vi "PH_SHS_Analysis.ProcCases.vi"(0 "i ref in":refnum<vi>, 1 "selector":string, 2 "Data":T2, 3 "call cluster":T3={"Object"="", "Selector"="", "CallType"=enum."synchronous", "Async Object"="", "Async Selector"="", "Data Descriptor"="", "Data"=[], "Error #"=0, "Expire"=0}, 5 "error in (no error)":errorcluster) -> (14 "i ref out":refnum<vi>, 17 "answer cluster":T3={"Object"="", "Selector"="", "CallType"=enum."synchronous", "Async Object"="", "Async Selector"="", "Data Descriptor"="", "Data"=[], "Error #"=0, "Expire"=0}, 19 "error out":errorcluster)   [LabVIEW 2014, in "PH_SHS_Analysis.lvlib"]
doc: "This method is called by a process from within the default case in the event loop. The methods of a class that are linked to events will be called from THIS method. Add your code here."
uses:
  PH_SHS_Analysis.lvlib
  CS_Core/CSSystem/CoreDefs/CoreDefs.call_type.ctl
  CS_Core/BaseProcess/BaseProcess.descriptor string definition.ctl
  CS_Core/CSSystem/CoreDefs/CoreDefs.rawDataType.ctl
  CSlibraries-extern/shs/SHS_Analysis/SHS_DeviceConfig.ctl
  CS_Core/CSSystem/CoreLib/CoreLib.string 2 byte array.vi
  CS_Core/CSSystem/CoreLib/CoreLib.byte array 2 short.vi
  CS_Core/CSSystem/CoreLib/CoreLib.byte array 2 string.vi
  CS_Core/CSSystem/CoreLib/CoreLib.byte array 2 double.vi
  CS_Core/BaseProcess/BaseProcess.lvlib
  CS_Core/CSSystem/CoreLib/CoreLib.lvlib
  CS_Core/CAEObj/CAEObj.lvlib
  PH_Basics/PH_PSDBWriter/PH_PSDBWriter.lvlib
  PH_Basics/PH_Common/PH_Common.lvlib
  CSlibraries-extern/shs/SHS_Analysis/SHS_Analysis.lvlib
  PH_Basics/PH_Img_BaseClass/PH_Img_BaseClass.lvlib
  PH_Basics/PH_Cam_BaseClass/PH_Cam_BaseClass.lvlib
panel:
  in  "SHS Device Config":T1 {"wavelength [m]" format="%#_6p"; "pixel size [m/px]" format="%#_6p"; "focal length [m]" format="%#_6p"}
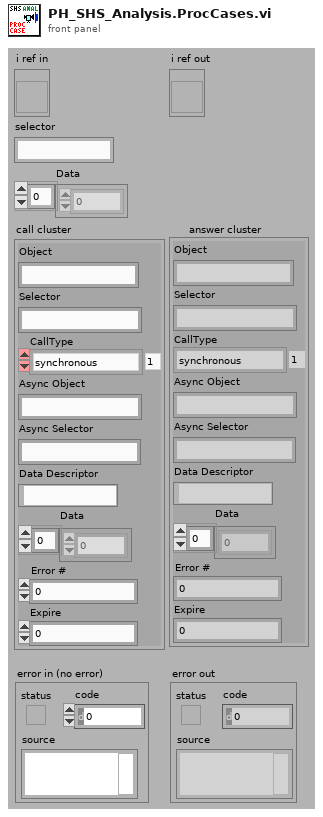
[diagram p1: front panel]
types:
  T1 = typedef "SHS_Analysis.lvlib/SHS_DeviceConfig.ctl" = cluster{"focal length [m]":dbl, "pixel size [m/px]":dbl, "wavelength [m]":dbl}
  T2 = typedef "CoreDefs.rawDataType.ctl" = i8[]
  T3 = typedef "CoreDefs.call_type.ctl" = cluster{"Object":string, "Selector":string, "CallType":enum16{"simple", "synchronous", "asynchronous"}, "Async Object":string, "Async Selector":string, "Data Descriptor":T4, "Data":T2, "Error #":i32, "Expire":u32}
  T4 = typedef "BaseProcess.lvlib/BaseProcess.descriptor string definition.ctl" = string
  T5 = cluster{"Cam ID":string, "Gain":dbl, "Brightness":dbl, "Shutter":dbl, "Cam Error":bool, "Mode":i32}
  T6 = enum8{"Enabled", "Disabled", "Disabled and Grayed Out"}
  T7 = typedef "PH_PSDBWriter.lvlib/PH_PSDBWriter.PHELIX-Subsystems.ctl" = i32
  T8 = typedef "PH_Cam_BaseClass.lvlib/PH_Cam_BaseClass.Settings.ctl" = cluster{"Cam ID":string, "Gain":dbl, "Brightness":dbl, "Shutter":dbl, "Mode":i32}
  T9 = typedef "PH_Img_BaseClass.lvlib/PH_Img_BaseClass.i attribute.ctl" = cluster{"GUI Refs":T10, "Timeout Image [ms]":i32, "Default Periodic Period [ms]":i32, "Camera":cluster{"Instancename":string, "Notifier":refnum<notifier>}, "Palette":T11, "Cam Settings":cluster{"Cam ID":string, "Gain":dbl, "Brightness":dbl, "Shutter":dbl, "Cam Info Failure":bool, "Mode":i32}}
  T10 = typedef "PH_Img_BaseClass.lvlib/PH_Img_BaseClass.GUI Refs.ctl" = cluster{"Timeout":refnum<vi>, "Image":refnum<vi>, "Palette":refnum<vi>, "Timeout Set":refnum<vi>}
  T11 = typedef "PH_Img_BaseClass.lvlib/PH_Img_BaseClass.Palette.ctl" = i32
  T12 = typedef "PH_SHS_Analysis.lvlib/PH_SHS_Analysis.i attribute.ctl" = cluster{"GUI Refs":cluster{"Delete":refnum<vi>, "Global On":refnum<vi>, "Cam Source":refnum<vi>, "Calibration Data File":refnum<vi>, "Calibration status":refnum<vi>, "Show overlay":refnum<vi>, "SHS Device Config":refnum<vi>, "Result":refnum<vi>, "Consider Tilt":refnum<vi>, "Working Reference":refnum<vi>, "Remove Tilt":refnum<vi>, "Take Cali  Reference":refnum<vi>, "Publishing Data Status":refnum<vi>, "Calibration Data":refnum<vi>}, "Calibration":cluster{"Status":T13, "Data":T14, "File":path}, "Result":T19, "Image":T22, "SHS Device Config":T1, "Show Overlay":bool, "GradientZernikeMatrix":dbl[][], "Consider Tilt":bool, "Working Reference":T15, "Zernicke Service ID":i32, "PSDB Image":T22}
  T13 = typedef "PH_StatusHandler.lvlib/PH_StatusHandler.Status.ctl" = i16
  T14 = typedef "PH_SHS_Analysis_Calibrator.lvlib/PH_SHS_Analysis_Calibrator.Analysis Calibration Data.ctl" = cluster{"Date":string, "Time":string, "Cam Settings":cluster{"Cam ID":string, "Gain":dbl, "Brightness":dbl, "Shutter":dbl, "Cam Error":bool, "Mode":i32}, "SHS Reference Result":T15, "Pixel Size":dbl, "MLA Pitch":dbl, "Method":enum16{"automatic", "manual"}, "Calibration Data calculated":bool, "No Problems at calculation?":bool, "error out":errorcluster}
  T15 = typedef "SHS_Common.lvlib/SHSReference.ctl" = cluster{"Reference":T16[][], "Lens Array Pitch [px]":dbl}
  T16 = typedef "SHS_Common.lvlib/ReferencePoint.ctl" = cluster{"Rect":T17, "Point":T18}
  T17 = typedef "SHS_Common.lvlib/Rectangle.ctl" = cluster{"Left":i32, "Top":i32, "Right":i32, "Bottom":i32}
  T18 = typedef "SHS_Common.lvlib/Point.ctl" = cluster{"x":dbl, "y":dbl, "valid?":bool, "weight":dbl}
  T19 = typedef "PH_SHS_Analysis.lvlib/PH_SHS_Analysis.Result.ctl" = cluster{"Time Stamp":timestamp, "Zernike Coefficients":T20, "PtV [lambda]":dbl, "Shifts":T21, "Measurement Quality":cluster{dbl, dbl, dbl}, "Measurement valid?":bool}
  T20 = typedef "PH_SHS_Analysis.lvlib/PH_SHS_Analysis.Zernike Coefficients.ctl" = cluster{"Tilt x":dbl, "Tilt y":dbl, "Defocus":dbl, "Astig 0°":dbl, "Astig 45°":dbl, "Coma x":dbl, "Coma y":dbl, "Spherical":dbl, "Trefoil 0°":dbl, "Trefoil 30°":dbl, "2nd Astig 0°":dbl, "2nd Astig 45°":dbl, "2nd Coma x":dbl, "2nd Coma y":dbl, "2nd Spherical":dbl}
  T21 = typedef "SHS_Common.lvlib/Shifts.ctl" = T18[][]
  T22 = typedef "IMAQ Image.ctl" = refnum<image>
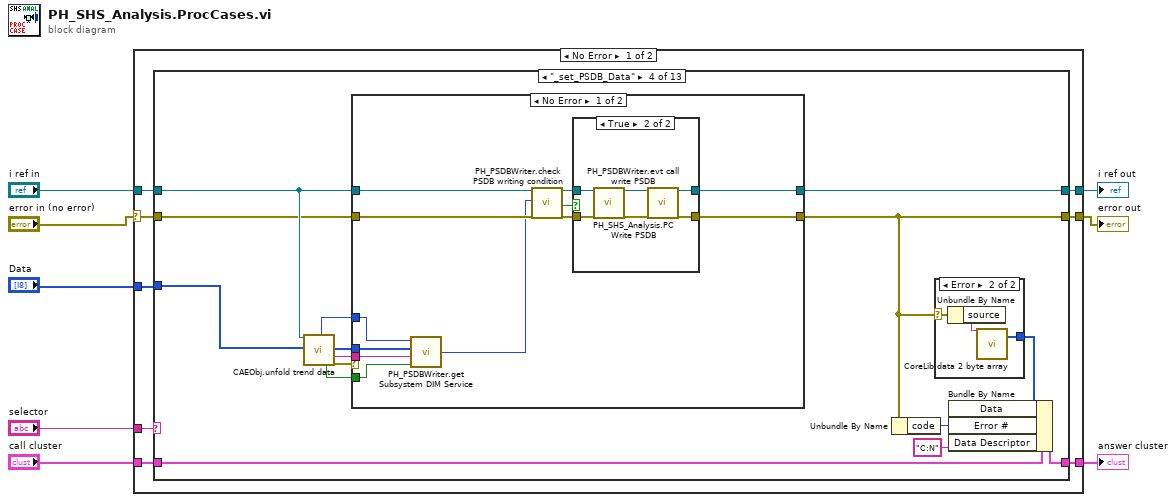
[diagram p0: block diagram]
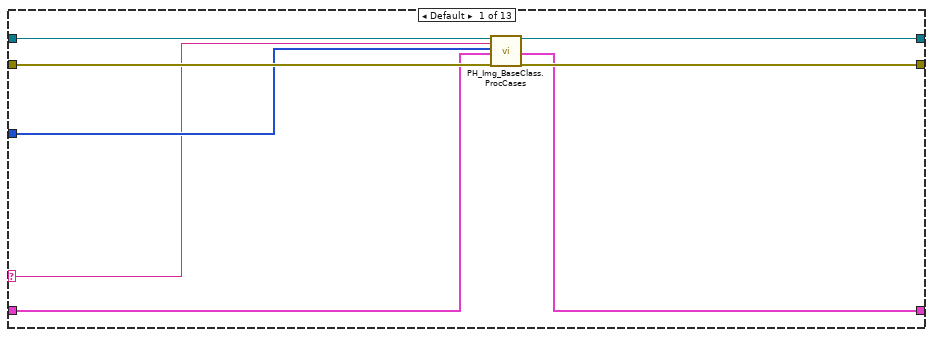
[diagram p2: hidden frame]
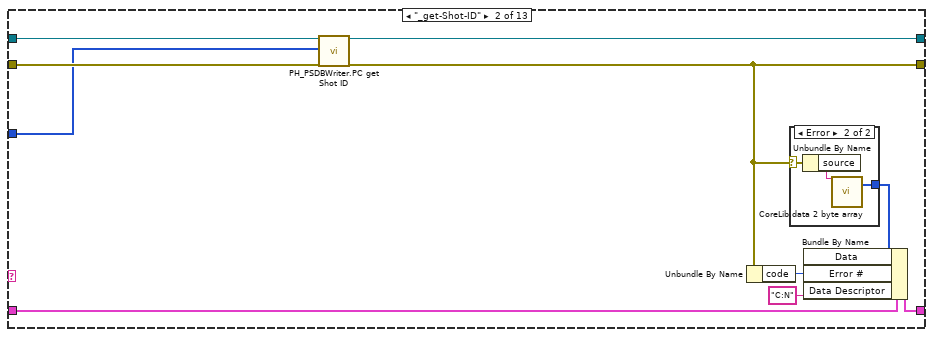
[diagram p3: hidden frame]
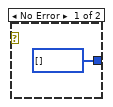
[diagram p4: hidden frame]
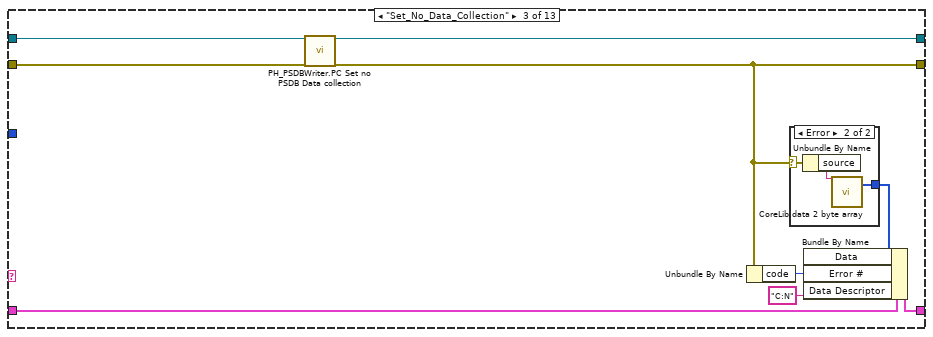
[diagram p5: hidden frame]
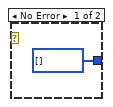
[diagram p6: hidden frame]
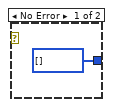
[diagram p9: hidden frame]
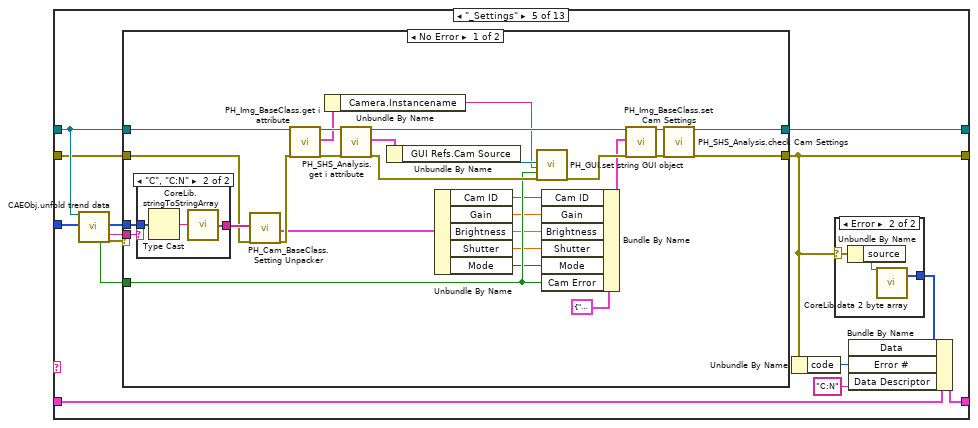
[diagram p10: hidden frame]
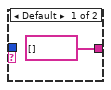
[diagram p11: hidden frame]
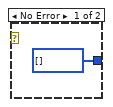
[diagram p13: hidden frame]
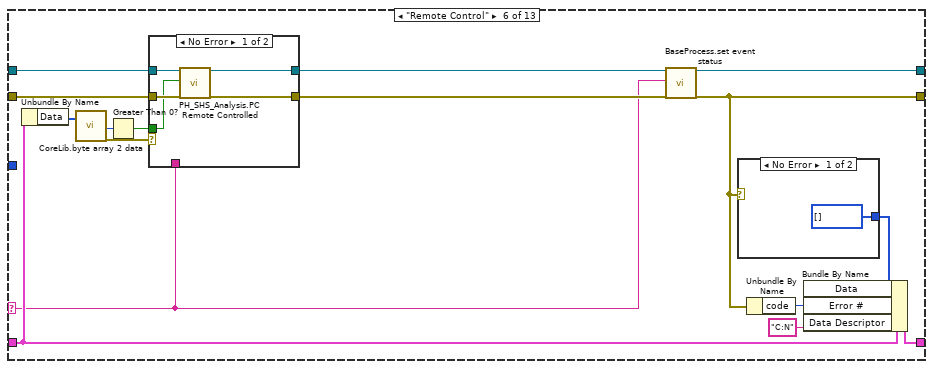
[diagram p14: hidden frame]
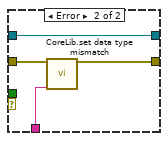
[diagram p15: hidden frame]
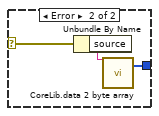
[diagram p16: hidden frame]
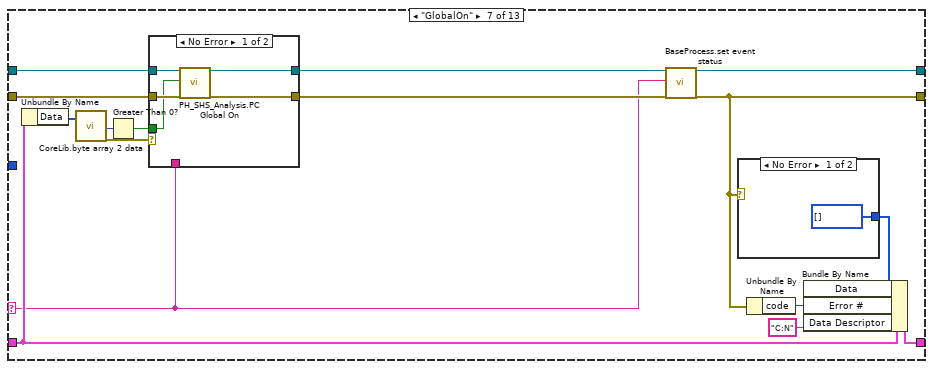
[diagram p17: hidden frame]
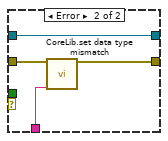
[diagram p18: hidden frame]
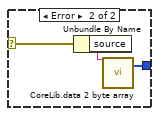
[diagram p19: hidden frame]
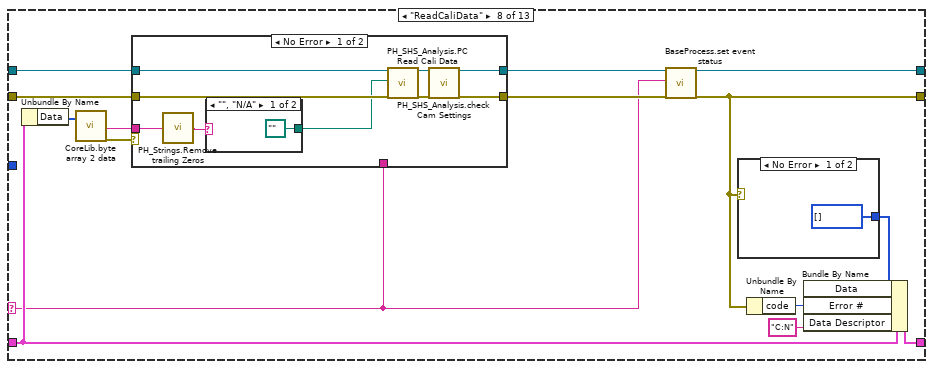
[diagram p20: hidden frame]
diagram:
  n1 = case shown="No Error" "error in (no error)" {
    selector: "error in (no error)" -> [w9 w456]
    tunnel: "selector" -> [w16 _]
    tunnel: [w15 w457] -> w7
    tunnel: "Data" -> [w14 _]
    tunnel: "call cluster" -> [w13 w457]
    tunnel: "i ref in" -> [w12 w458]
    tunnel: [w11 w458] -> w3
    tunnel: [w10 w456] -> w2
    frame No Error {
      n2 = case shown="\"_set_PSDB_Data\"" w16 {
        selector: w16 -> [w18 _ _ _ _ w145 w174 w204 w246 w293 w330 w374 w425]
        tunnel: w14 -> [w19 w25 _ w52 w97 _ _ _ _ _ _ _ _]
        tunnel: w12 -> [w17 w29 w41 w56 w96 w149 w178 w208 w245 w292 w335 w379 w430]
        tunnel: [w24 w27 w40 w54 w94 w156 w185 w213 w249 w296 w340 w384 w434] -> w11
        tunnel: w13 -> [w20 w33 w46 w65 w105 w148 w177 w207 w247 w294 w331 w375 w426]
        tunnel: [w21 w32 w45 w64 w104 w159 w188 w216 w252 w299 w343 w387 w437] -> w15
        tunnel: w9 -> [w23 w28 w42 w55 w95 w150 w179 w209 w244 w291 w334 w378 w429]
        tunnel: [w22 w26 w39 w53 w93 w157 w186 w214 w250 w297 w341 w385 w435] -> w10
        frame Default {
          n3 = call "PH_Img_BaseClass.ProcCases.vi"("i ref in"=w17, "selector"=w18, "Data"=w19, "call cluster"=w20, "error in (no error)"=w23) -> ("i ref out"=w24:refnum<vi>, "answer cluster"=w21:T3, "error out"=w22:errorcluster)  [unwired: 12 in]
        }
        frame "_get-Shot-ID" {
          n4 = call "PH_PSDBWriter.PC get Shot ID.vi"("i ref in"=w29, "Data"=w25, "error IO"=w28) -> ("i ref in"=w27:refnum<vi>, "error IO"=w26:errorcluster)  [unwired: 15 in]
          n5 = Unbundle By Name(w26) -> ("code"=w34:i32)
          n6 = case shown="Error" w26 {
            selector: w26 -> [_ w38]
            tunnel: [T2 [] ("byteArray out") w37] -> w31
            frame No Error {
            }
            frame Error {
              n7 = Unbundle By Name(w38) -> ("source"=w36:string)
              n8 = call-poly "CoreLib.data 2 byte array.vi"("string"=w36) -> ("byteArray out"=w37:T2)  [unwired: 18 in]
            }
          }
          n9 = Bundle By Name(cluster=w33, "Data"=w31, "Error #"=w34, "Data Descriptor"="C:N") -> (w32:T3)
        }
        frame "Set_No_Data_Collection" {
          n10 = call "PH_PSDBWriter.PC Set no PSDB Data collection.vi"("i ref in"=w41, "error IO"=w42) -> ("i ref out"=w40:refnum<vi>, "error out"=w39:errorcluster)  [unwired: 16 in]
          n11 = Unbundle By Name(w39) -> ("code"=w47:i32)
          n12 = case shown="Error" w39 {
            selector: w39 -> [_ w51]
            tunnel: [T2 [] ("byteArray out") w50] -> w44
            frame No Error {
            }
            frame Error {
              n13 = Unbundle By Name(w51) -> ("source"=w49:string)
              n14 = call-poly "CoreLib.data 2 byte array.vi"("string"=w49) -> ("byteArray out"=w50:T2)  [unwired: 18 in]
            }
          }
          n15 = Bundle By Name(cluster=w46, "Data"=w44, "Error #"=w47, "Data Descriptor"="C:N") -> (w45:T3)
        }
        frame "_set_PSDB_Data" {
          n16 = call "CAEObj.unfold trend data.vi"("i ref in"=w56, "raw trend data"=w52) -> ("quality"=w57:i32, "no link"=w60:bool, "data"=w58:i8[], "typeDescriptor"=w59:string, "error out"=w61:errorcluster)  [unwired: 9 in, 4 out]
          n17 = case shown="No Error" w61 {
            tunnel: w55 -> [w78 w88]
            tunnel: [w77 w87] -> w54
            tunnel: [w76 w88] -> w53
            tunnel: w56 -> [w74 w87]
            tunnel: w60 -> [w68 _]
            tunnel: w59 -> [w70 _]
            tunnel: w58 -> [w71 _]
            tunnel: w57 -> [w69 _]
            frame No Error {
              n18 = call "PH_PSDBWriter.get Subsystem DIM Service.vi"("no link"=w68, "typeDescriptor"=w70, "data"=w71, "quality"=w69) -> ("PHELIX Subsystems"=w67:T7)
              n19 = call "PH_PSDBWriter.check PSDB writing condition.vi"("i ref in"=w74, "wanted Subsystem"=w67, "error IO"=w78) -> ("i ref out"=w73:refnum<vi>, "write PSDB?"=w72:bool, "error out"=w75:errorcluster)  [unwired: 14 in]
              n20 = case shown="True" w72 {
                tunnel: w75 -> [w79 w86]
                tunnel: [w80 w83] -> w77
                tunnel: [w79 w81] -> w76
                tunnel: w73 -> [w80 w85]
                frame False {
                }
                frame True {
                  n21 = call "PH_SHS_Analysis.PC Write PSDB.vi"("i ref in"=w85, "error IO"=w86) -> ("i ref out"=w84:refnum<vi>, "error out"=w82:errorcluster)  [unwired: 16 in]
                  n22 = call "PH_PSDBWriter.evt call write PSDB.vi"("i ref in"=w84, "error in (no error)"=w82) -> ("i ref out"=w83:refnum<vi>, "error out"=w81:errorcluster)  [unwired: 16 in]
                }
              }
            }
            frame Error {
            }
          }
          n23 = Unbundle By Name(w53) -> ("code"=w66:i32)
          n24 = case shown="Error" w53 {
            selector: w53 -> [_ w92]
            tunnel: [T2 [] ("byteArray out") w91] -> w63
            frame No Error {
            }
            frame Error {
              n25 = Unbundle By Name(w92) -> ("source"=w90:string)
              n26 = call-poly "CoreLib.data 2 byte array.vi"("string"=w90) -> ("byteArray out"=w91:T2)  [unwired: 18 in]
            }
          }
          n27 = Bundle By Name(cluster=w65, "Data"=w63, "Error #"=w66, "Data Descriptor"="C:N") -> (w64:T3)
        }
        frame "_Settings" {
          n28 = call "CAEObj.unfold trend data.vi"("i ref in"=w96, "raw trend data"=w97) -> ("no link"=w98:bool, "data"=w99:i8[], "typeDescriptor"=w100:string, "error out"=w101:errorcluster)  [unwired: 9 in, 5 out]
          n29 = case shown="No Error" w101 {
            tunnel: w96 -> [w119 w140]
            tunnel: [w121 w140] -> w94
            tunnel: w95 -> [w131 w139]
            tunnel: [w123 w139] -> w93
            tunnel: w100 -> [w134 _]
            tunnel: w99 -> [w133 _]
            tunnel: w98 -> [w124 _]
            frame No Error {
              n30 = case shown="\"C\", \"C:N\"" w134 {
                tunnel: w133 -> [_ w138]
                tunnel: [string[] [] ("Array") w136] -> w132
                frame Default {
                }
                frame "C", "C:N" {
                  n31 = Type Cast(x=w138) -> (*(type *) &x=w137:string)  [unwired: 1 in]
                  n32 = call "CoreLib.stringToStringArray.vi"("String"=w137) -> ("Array"=w136:string[])
                }
              }
              n33 = call "PH_Cam_BaseClass.Setting Unpacker.vi"("Cam Settings Array"=w132, "error in (no error)"=w131) -> ("Cam Settings"=w126:T8, "error out"=w130:errorcluster)  [unwired: 15 in, 1 out]
              n34 = call "PH_Img_BaseClass.get i attribute.vi"("i ref in"=w119, "error in (no error)"=w130) -> ("i ref out"=w118:refnum<vi>, "i attribute"=w117:T9, "error out"=w120:errorcluster)  [unwired: 15 in]
              n35 = Unbundle By Name(w117) -> ("Camera.Instancename"=w107:string)
              n36 = call "PH_SHS_Analysis.get i attribute.vi"("i ref in"=w118, "error in (no error)"=w120) -> ("i ref out"=w127:refnum<vi>, "i attribute"=w125:T12, "error out"=w129:errorcluster)  [unwired: 15 in]
              n37 = Unbundle By Name(w125) -> ("GUI Refs.Cam Source"=w111:refnum<vi>)
              n38 = Unbundle By Name(w126) -> ("Cam ID"=w108:string, "Gain"=w116:dbl, "Brightness"=w115:dbl, "Shutter"=w114:dbl, "Mode"=w113:i32)
              n39 = call "PH_GUI.set string GUI object.vi"("GUI object Ref"=w111, "Text"=w107, "Blinking? (false)"=w124, "error in"=w129) -> ("error out"=w112:errorcluster)  [unwired: 15 in]
              n40 = Bundle By Name(cluster=T5 {"Cam ID"="N/A", "Gain"=nan, "Brightness"=nan, "Shutter"=nan, "Cam Error"=TRUE, "Mode"=-1} ("Cam Settings"), "Cam ID"=w108, "Gain"=w116, "Brightness"=w115, "Shutter"=w114, "Mode"=w113, "Cam Error"=w124) -> (w109:T5)
              n41 = call "PH_Img_BaseClass.set Cam Settings.vi"("i ref in"=w127, "Cam Settings"=w109, "error in (no error)"=w112) -> ("i ref out"=w122:refnum<vi>, "error out"=w128:errorcluster)  [unwired: 15 in]
              n42 = call "PH_SHS_Analysis.check Cam Settings.vi"("i ref in"=w122, "error in"=w128) -> ("i ref out"=w121:refnum<vi>, "error out"=w123:errorcluster)  [unwired: 16 in]
            }
            frame Error {
            }
          }
          n43 = Unbundle By Name(w93) -> ("code"=w106:i32)
          n44 = case shown="Error" w93 {
            selector: w93 -> [_ w144]
            tunnel: [T2 [] ("byteArray out") w143] -> w103
            frame No Error {
            }
            frame Error {
              n45 = Unbundle By Name(w144) -> ("source"=w142:string)
              n46 = call-poly "CoreLib.data 2 byte array.vi"("string"=w142) -> ("byteArray out"=w143:T2)  [unwired: 18 in]
            }
          }
          n47 = Bundle By Name(cluster=w105, "Data"=w103, "Error #"=w106, "Data Descriptor"="C:N") -> (w104:T3)
        }
        frame "Remote Control" {
          n48 = Unbundle By Name(w148) -> ("Data"=w151:T2)
          n49 = call-poly "CoreLib.byte array 2 data.vi"("byteArray"=w151) -> ("i16"=w152:i16, "error out"=w154:errorcluster)  [unwired: 16 in, 1 out]
          n50 = Greater Than 0?(x=w152) -> (x > 0?=w153:bool)
          n51 = case shown="No Error" w154 {
            tunnel: [w162 w169] -> w147
            tunnel: w149 -> [w164 w169]
            tunnel: w150 -> [w163 w168]
            tunnel: [w165 w167] -> w146
            tunnel: w145 -> [_ w166]
            tunnel: w153 -> [w161 _]
            frame No Error {
              n52 = call "PH_SHS_Analysis.PC Remote Controlled.vi"("i ref in"=w164, "Remote Controlled?"=w161, "error in (no error)"=w163) -> ("i ref out"=w162:refnum<vi>, "error out"=w165:errorcluster)  [unwired: 15 in]
            }
            frame Error {
              n53 = call "CoreLib.set data type mismatch.vi"("error in (no error)"=w168, "error source"=w166) -> ("error out"=w167:errorcluster)  [unwired: 17 in]
            }
          }
          n54 = call "BaseProcess.set event status.vi"("i ref in"=w147, "EventStatus"=w145, "error in (no error)"=w146) -> ("i ref out"=w156:refnum<vi>, "error out"=w157:errorcluster)  [unwired: 14 in, 1 out]
          n55 = case shown="No Error" w157 {
            selector: w157 -> [_ w173]
            tunnel: [T2 [] ("byteArray out") w172] -> w158
            frame No Error {
            }
            frame Error {
              n56 = Unbundle By Name(w173) -> ("source"=w171:string)
              n57 = call-poly "CoreLib.data 2 byte array.vi"("string"=w171) -> ("byteArray out"=w172:T2)  [unwired: 18 in]
            }
          }
          n58 = Unbundle By Name(w157) -> ("code"=w160:i32)
          n59 = Bundle By Name(cluster=w148, "Data"=w158, "Error #"=w160, "Data Descriptor"="C:N") -> (w159:T3)
        }
        frame "GlobalOn" {
          n60 = Unbundle By Name(w177) -> ("Data"=w180:T2)
          n61 = call-poly "CoreLib.byte array 2 data.vi"("byteArray"=w180) -> ("i16"=w181:i16, "error out"=w183:errorcluster)  [unwired: 16 in, 1 out]
          n62 = Greater Than 0?(x=w181) -> (x > 0?=w182:bool)
          n63 = case shown="No Error" w183 {
            tunnel: [w191 w198] -> w176
            tunnel: w178 -> [w193 w198]
            tunnel: w179 -> [w192 w197]
            tunnel: [w194 w196] -> w175
            tunnel: w174 -> [_ w195]
            tunnel: w182 -> [w190 _]
            frame No Error {
              n64 = call "PH_SHS_Analysis.PC Global On.vi"("i ref in"=w193, "Global On?"=w190, "error in (no error)"=w192) -> ("i ref out"=w191:refnum<vi>, "error out"=w194:errorcluster)  [unwired: 15 in]
            }
            frame Error {
              n65 = call "CoreLib.set data type mismatch.vi"("error in (no error)"=w197, "error source"=w195) -> ("error out"=w196:errorcluster)  [unwired: 17 in]
            }
          }
          n66 = call "BaseProcess.set event status.vi"("i ref in"=w176, "EventStatus"=w174, "error in (no error)"=w175) -> ("i ref out"=w185:refnum<vi>, "error out"=w186:errorcluster)  [unwired: 14 in, 1 out]
          n67 = case shown="No Error" w186 {
            selector: w186 -> [_ w202]
            tunnel: [T2 [] ("byteArray out") w201] -> w187
            frame No Error {
            }
            frame Error {
              n68 = Unbundle By Name(w202) -> ("source"=w200:string)
              n69 = call-poly "CoreLib.data 2 byte array.vi"("string"=w200) -> ("byteArray out"=w201:T2)  [unwired: 18 in]
            }
          }
          n70 = Unbundle By Name(w186) -> ("code"=w189:i32)
          n71 = Bundle By Name(cluster=w177, "Data"=w187, "Error #"=w189, "Data Descriptor"="C:N") -> (w188:T3)
        }
        frame "ReadCaliData" {
          n72 = Unbundle By Name(w207) -> ("Data"=w210:T2)
          n73 = call-poly "CoreLib.byte array 2 data.vi"("byteArray"=w210) -> ("string"=w203:string, "error out"=w211:errorcluster)  [unwired: 16 in, 1 out]
          n74 = case shown="No Error" w211 {
            tunnel: [w220 w233] -> w206
            tunnel: w208 -> [w226 w233]
            tunnel: w209 -> [w225 w232]
            tunnel: [w218 w231] -> w205
            tunnel: w204 -> [_ w230]
            tunnel: w203 -> [w224 _]
            frame No Error {
              n75 = call "PH_Strings.Remove trailing Zeros.vi"("Input String"=w224) -> ("Output String"=w222:string)
              n76 = case shown="\"\", \"N/A\"" w222 {
                selector: w222 -> [_ w228]
                tunnel: [path "" w229] -> w223
                frame "", "N/A" {
                }
                frame Default {
                  n77 = String To Path(string=w228) -> (path=w229:path)
                }
              }
              n78 = call "PH_SHS_Analysis.PC Read Cali Data.vi"("i ref in"=w226, "Cali Data File"=w223, "error in (no error)"=w225) -> ("i ref out"=w221:refnum<vi>, "error out"=w219:errorcluster)  [unwired: 15 in]
              n79 = call "PH_SHS_Analysis.check Cam Settings.vi"("i ref in"=w221, "error in"=w219) -> ("i ref out"=w220:refnum<vi>, "error out"=w218:errorcluster)  [unwired: 16 in]
            }
            frame Error {
              n80 = call "CoreLib.set data type mismatch.vi"("error in (no error)"=w232, "error source"=w230) -> ("error out"=w231:errorcluster)  [unwired: 17 in]
            }
          }
          n81 = call "BaseProcess.set event status.vi"("i ref in"=w206, "EventStatus"=w204, "error in (no error)"=w205) -> ("i ref out"=w213:refnum<vi>, "error out"=w214:errorcluster)  [unwired: 14 in, 1 out]
          n82 = case shown="No Error" w214 {
            selector: w214 -> [_ w237]
            tunnel: [T2 [] ("byteArray out") w236] -> w215
            frame No Error {
            }
            frame Error {
              n83 = Unbundle By Name(w237) -> ("source"=w235:string)
              n84 = call-poly "CoreLib.data 2 byte array.vi"("string"=w235) -> ("byteArray out"=w236:T2)  [unwired: 18 in]
            }
          }
          n85 = Unbundle By Name(w214) -> ("code"=w217:i32)
          n86 = Bundle By Name(cluster=w207, "Data"=w215, "Error #"=w217, "Data Descriptor"="C:N") -> (w216:T3)
        }
        frame "RemoveTilt" {
          n87 = call "PH_SHS_Analysis.get data to modify.vi"("i ref in"=w245, "error in (no error)"=w244) -> ("i ref out"=w243:refnum<vi>, "i attribute"=w238:T12, "timed out"=w239:bool, "error out"=w241:errorcluster)  [unwired: 14 in]
          n88 = case shown="False" w239 {
            tunnel: w243 -> [w268 w280]
            tunnel: [w267 w280] -> w242
            tunnel: w241 -> [w255 w279]
            tunnel: [w266 w279] -> w240
            tunnel: w238 -> [w264 _]
            frame False {
              n89 = Unbundle By Name(w264) -> ("GUI Refs.Take Cali  Reference"=w256:refnum<vi>, "GUI Refs.Working Reference"=w258:refnum<vi>, "Working Reference"=w263:T15, "Result.Shifts"=w262:T21)
              n90 = Not A Number/Path/Refnum?(number/path/refnum=w256) -> (NaN/Path/Refnum?=w257:bool)
              n91 = case shown="False" w257 {
                tunnel: w255 -> [w272 w273]
                tunnel: [w271 w273] -> w254
                tunnel: w256 -> [w270 _]
                frame False {
                  n92 = property class="Bool"(reference=w270, error in=w272, "DisabledEnum"=T6."Enabled" ("Disabled")) -> (error out=w271:errorcluster)  [unwired: 1 out]
                }
                frame True {
                }
              }
              n93 = call "RemoveTilt.vi"("SHS Reference"=w263, "Shifts"=w262) -> ("tilt corrected SHS Reference"=w260:T15)  [unwired: 17 in]
              n94 = Not A Number/Path/Refnum?(number/path/refnum=w258) -> (NaN/Path/Refnum?=w259:bool)
              n95 = case shown="False" w259 {
                tunnel: w254 -> [w277 w278]
                tunnel: [w276 w278] -> w261
                tunnel: w258 -> [w275 _]
                tunnel: w260 -> [w274 _]
                frame False {
                  n96 = property class="Clust (strict)"(reference=w275, error in=w277, "Value"=w274) -> (error out=w276:errorcluster)  [unwired: 1 out]
                }
                frame True {
                }
              }
              n97 = Bundle By Name(cluster=w264, "Working Reference"=w260) -> (w265:T12)
              n98 = call "PH_SHS_Analysis.set modified data.vi"("i ref in"=w268, "i attribute"=w265, "error in (no error)"=w261) -> ("i ref out"=w267:refnum<vi>, "error out"=w266:errorcluster)  [unwired: 15 in]
            }
            frame True {
            }
          }
          n99 = call "BaseProcess.set event status.vi"("i ref in"=w242, "EventStatus"=w246, "error in (no error)"=w240) -> ("i ref out"=w249:refnum<vi>, "error out"=w250:errorcluster)  [unwired: 14 in, 1 out]
          n100 = Unbundle By Name(w250) -> ("code"=w253:i32)
          n101 = case shown="No Error" w250 {
            selector: w250 -> [_ w284]
            tunnel: [T2 [] ("byteArray out") w283] -> w251
            frame No Error {
            }
            frame Error {
              n102 = Unbundle By Name(w284) -> ("source"=w282:string)
              n103 = call-poly "CoreLib.data 2 byte array.vi"("string"=w282) -> ("byteArray out"=w283:T2)  [unwired: 18 in]
            }
          }
          n104 = Bundle By Name(cluster=w247, "Data"=w251, "Error #"=w253, "Data Descriptor"="C:N") -> (w252:T3)
        }
        frame "TakeCaliRef" {
          n105 = call "PH_SHS_Analysis.get data to modify.vi"("i ref in"=w292, "error in (no error)"=w291) -> ("i ref out"=w290:refnum<vi>, "i attribute"=w285:T12, "timed out"=w286:bool, "error out"=w288:errorcluster)  [unwired: 14 in]
          n106 = case shown="False" w286 {
            tunnel: w290 -> [w313 w325]
            tunnel: [w312 w325] -> w289
            tunnel: w288 -> [w302 w324]
            tunnel: [w311 w324] -> w287
            tunnel: w285 -> [w309 _]
            frame False {
              n107 = Unbundle By Name(w309) -> ("GUI Refs.Take Cali  Reference"=w301:refnum<vi>, "GUI Refs.Working Reference"=w306:refnum<vi>, "Calibration.Data.SHS Reference Result"=w305:T15)
              n108 = Not A Number/Path/Refnum?(number/path/refnum=w301) -> (NaN/Path/Refnum?=w304:bool)
              n109 = case shown="False" w304 {
                tunnel: w302 -> [w317 w318]
                tunnel: [w316 w318] -> w303
                tunnel: w301 -> [w315 _]
                frame False {
                  n110 = property class="Bool"(reference=w315, error in=w317, "DisabledEnum"=T6."Disabled and Grayed Out" ("Disabled")) -> (error out=w316:errorcluster)  [unwired: 1 out]
                }
                frame True {
                }
              }
              n111 = Not A Number/Path/Refnum?(number/path/refnum=w306) -> (NaN/Path/Refnum?=w307:bool)
              n112 = case shown="False" w307 {
                tunnel: w303 -> [w322 w323]
                tunnel: [w321 w323] -> w308
                tunnel: w306 -> [w320 _]
                tunnel: w305 -> [w319 _]
                frame False {
                  n113 = property class="Clust (strict)"(reference=w320, error in=w322, "Value"=w319) -> (error out=w321:errorcluster)  [unwired: 1 out]
                }
                frame True {
                }
              }
              n114 = Bundle By Name(cluster=w309, "Working Reference"=w305) -> (w310:T12)
              n115 = call "PH_SHS_Analysis.set modified data.vi"("i ref in"=w313, "i attribute"=w310, "error in (no error)"=w308) -> ("i ref out"=w312:refnum<vi>, "error out"=w311:errorcluster)  [unwired: 15 in]
            }
            frame True {
            }
          }
          n116 = call "BaseProcess.set event status.vi"("i ref in"=w289, "EventStatus"=w293, "error in (no error)"=w287) -> ("i ref out"=w296:refnum<vi>, "error out"=w297:errorcluster)  [unwired: 14 in, 1 out]
          n117 = Unbundle By Name(w297) -> ("code"=w300:i32)
          n118 = case shown="No Error" w297 {
            selector: w297 -> [_ w329]
            tunnel: [T2 [] ("byteArray out") w328] -> w298
            frame No Error {
            }
            frame Error {
              n119 = Unbundle By Name(w329) -> ("source"=w327:string)
              n120 = call-poly "CoreLib.data 2 byte array.vi"("string"=w327) -> ("byteArray out"=w328:T2)  [unwired: 18 in]
            }
          }
          n121 = Bundle By Name(cluster=w294, "Data"=w298, "Error #"=w300, "Data Descriptor"="C:N") -> (w299:T3)
        }
        frame "ShowOverlay" {
          n122 = Unbundle By Name(w331) -> ("Data"=w338:T2)
          n123 = call-poly "CoreLib.byte array 2 data.vi"("byteArray"=w338) -> ("i16"=w336:i16, "error out"=w337:errorcluster)  [unwired: 16 in, 1 out]
          n124 = case shown="No Error" w337 {
            tunnel: [w351 w369] -> w332
            tunnel: w335 -> [w352 w369]
            tunnel: w334 -> [w350 w368]
            tunnel: [w349 w367] -> w333
            tunnel: w336 -> [w346 _]
            tunnel: w330 -> [_ w366]
            frame No Error {
              n125 = call "PH_SHS_Analysis.get data to modify.vi"("i ref in"=w352, "error in (no error)"=w350) -> ("i ref out"=w353:refnum<vi>, "i attribute"=w347:T12, "timed out"=w348:bool, "error out"=w354:errorcluster)  [unwired: 14 in]
              n126 = Greater Than 0?(x=w346) -> (x > 0?=w345:bool)
              n127 = case shown="False" w348 {
                tunnel: w354 -> [w358 w364]
                tunnel: w353 -> [w363 w365]
                tunnel: [w362 w365] -> w351
                tunnel: [w361 w364] -> w349
                tunnel: w347 -> [w359 _]
                tunnel: w345 -> [w355 _]
                frame False {
                  n128 = Unbundle By Name(w359) -> ("GUI Refs.Show overlay"=w356:refnum<vi>)
                  n129 = call "PH_GUI.set boolean GUI object.vi"("Boolean Knob GUI Ref"=w356, "Value"=w355, "error in (no error)"=w358) -> ("error out"=w357:errorcluster)  [unwired: 16 in]
                  n130 = Bundle By Name(cluster=w359, "Show Overlay"=w355) -> (w360:T12)
                  n131 = call "PH_SHS_Analysis.set modified data.vi"("i ref in"=w363, "i attribute"=w360, "error in (no error)"=w357) -> ("i ref out"=w362:refnum<vi>, "error out"=w361:errorcluster)  [unwired: 15 in]
                }
                frame True {
                }
              }
            }
            frame Error {
              n132 = call "CoreLib.set data type mismatch.vi"("error in (no error)"=w368, "error source"=w366) -> ("error out"=w367:errorcluster)  [unwired: 17 in]
            }
          }
          n133 = call "BaseProcess.set event status.vi"("i ref in"=w332, "EventStatus"=w330, "error in (no error)"=w333) -> ("i ref out"=w340:refnum<vi>, "error out"=w341:errorcluster)  [unwired: 14 in, 1 out]
          n134 = Unbundle By Name(w341) -> ("code"=w344:i32)
          n135 = case shown="No Error" w341 {
            selector: w341 -> [_ w373]
            tunnel: [T2 [] ("byteArray out") w372] -> w342
            frame No Error {
            }
            frame Error {
              n136 = Unbundle By Name(w373) -> ("source"=w371:string)
              n137 = call-poly "CoreLib.data 2 byte array.vi"("string"=w371) -> ("byteArray out"=w372:T2)  [unwired: 18 in]
            }
          }
          n138 = Bundle By Name(cluster=w331, "Data"=w342, "Error #"=w344, "Data Descriptor"="C:N") -> (w343:T3)
        }
        frame "ConsiderTilt" {
          n139 = Unbundle By Name(w375) -> ("Data"=w382:T2)
          n140 = call-poly "CoreLib.byte array 2 data.vi"("byteArray"=w382) -> ("i16"=w380:i16, "error out"=w381:errorcluster)  [unwired: 16 in, 1 out]
          n141 = case shown="No Error" w381 {
            tunnel: [w395 w413] -> w376
            tunnel: w379 -> [w396 w413]
            tunnel: w378 -> [w394 w412]
            tunnel: [w393 w411] -> w377
            tunnel: w380 -> [w390 _]
            tunnel: w374 -> [_ w410]
            frame No Error {
              n142 = call "PH_SHS_Analysis.get data to modify.vi"("i ref in"=w396, "error in (no error)"=w394) -> ("i ref out"=w397:refnum<vi>, "i attribute"=w391:T12, "timed out"=w392:bool, "error out"=w398:errorcluster)  [unwired: 14 in]
              n143 = Greater Than 0?(x=w390) -> (x > 0?=w389:bool)
              n144 = case shown="False" w392 {
                tunnel: w398 -> [w402 w408]
                tunnel: w397 -> [w407 w409]
                tunnel: [w406 w409] -> w395
                tunnel: [w405 w408] -> w393
                tunnel: w391 -> [w403 _]
                tunnel: w389 -> [w399 _]
                frame False {
                  n145 = Unbundle By Name(w403) -> ("GUI Refs.Consider Tilt"=w400:refnum<vi>)
                  n146 = call "PH_GUI.set boolean GUI object.vi"("Boolean Knob GUI Ref"=w400, "Value"=w399, "error in (no error)"=w402) -> ("error out"=w401:errorcluster)  [unwired: 16 in]
                  n147 = Bundle By Name(cluster=w403, "Consider Tilt"=w399) -> (w404:T12)
                  n148 = call "PH_SHS_Analysis.set modified data.vi"("i ref in"=w407, "i attribute"=w404, "error in (no error)"=w401) -> ("i ref out"=w406:refnum<vi>, "error out"=w405:errorcluster)  [unwired: 15 in]
                }
                frame True {
                }
              }
            }
            frame Error {
              n149 = call "CoreLib.set data type mismatch.vi"("error in (no error)"=w412, "error source"=w410) -> ("error out"=w411:errorcluster)  [unwired: 17 in]
            }
          }
          n150 = call "BaseProcess.set event status.vi"("i ref in"=w376, "EventStatus"=w374, "error in (no error)"=w377) -> ("i ref out"=w384:refnum<vi>, "error out"=w385:errorcluster)  [unwired: 14 in, 1 out]
          n151 = Unbundle By Name(w385) -> ("code"=w388:i32)
          n152 = case shown="No Error" w385 {
            selector: w385 -> [_ w417]
            tunnel: [T2 [] ("byteArray out") w416] -> w386
            frame No Error {
            }
            frame Error {
              n153 = Unbundle By Name(w417) -> ("source"=w415:string)
              n154 = call-poly "CoreLib.data 2 byte array.vi"("string"=w415) -> ("byteArray out"=w416:T2)  [unwired: 18 in]
            }
          }
          n155 = Bundle By Name(cluster=w375, "Data"=w386, "Error #"=w388, "Data Descriptor"="C:N") -> (w387:T3)
        }
        frame "SetSHSDevConfig" {
          n156 = Unbundle By Name(w426) -> ("Data"=w432:T2)
          n157 = call-poly "CoreLib.byte array 2 data.vi"("byteArray"=w432) -> ("byteArray out"=w419:T2, "d64"=w431:dbl, "error out"=w423:errorcluster)  [unwired: 16 in]
          n158 = call-poly "CoreLib.byte array 2 data.vi"("byteArray"=w419, "error in (no error)"=w423) -> ("byteArray out"=w418:T2, "d64"=w421:dbl, "error out"=w424:errorcluster)  [unwired: 15 in]
          n159 = call-poly "CoreLib.byte array 2 data.vi"("byteArray"=w418, "error in (no error)"=w424) -> ("d64"=w420:dbl, "error out"=w422:errorcluster)  [unwired: 15 in, 1 out]
          n160 = case shown="No Error" w422 {
            tunnel: [w446 w451] -> w427
            tunnel: w430 -> [w447 w451]
            tunnel: w429 -> [w445 w450]
            tunnel: [w444 w449] -> w428
            tunnel: w431 -> [w441 _]
            tunnel: w425 -> [_ w448]
            tunnel: w421 -> [w440 _]
            tunnel: w420 -> [w439 _]
            frame No Error {
              n161 = Bundle By Name(cluster="SHS Device Config", "focal length [m]"=w441, "pixel size [m/px]"=w440, "wavelength [m]"=w439) -> (w443:T1)
              n162 = call "PH_SHS_Analysis.PC Set SHS Device Config.vi"("i ref in"=w447, "SHS Device Config"=w443, "error IO"=w445) -> ("i ref out"=w446:refnum<vi>, "error out"=w444:errorcluster)  [unwired: 15 in]
            }
            frame Error {
              n163 = call "CoreLib.set data type mismatch.vi"("error in (no error)"=w450, "error source"=w448) -> ("error out"=w449:errorcluster)  [unwired: 17 in]
            }
          }
          n164 = call "BaseProcess.set event status.vi"("i ref in"=w427, "EventStatus"=w425, "error in (no error)"=w428) -> ("i ref out"=w434:refnum<vi>, "error out"=w435:errorcluster)  [unwired: 14 in, 1 out]
          n165 = Unbundle By Name(w435) -> ("code"=w438:i32)
          n166 = case shown="No Error" w435 {
            selector: w435 -> [_ w455]
            tunnel: [T2 [] ("byteArray out") w454] -> w436
            frame No Error {
            }
            frame Error {
              n167 = Unbundle By Name(w455) -> ("source"=w453:string)
              n168 = call-poly "CoreLib.data 2 byte array.vi"("string"=w453) -> ("byteArray out"=w454:T2)  [unwired: 18 in]
            }
          }
          n169 = Bundle By Name(cluster=w426, "Data"=w436, "Error #"=w438, "Data Descriptor"="C:N") -> (w437:T3)
        }
      }
    }
    frame Error {
    }
  }
  "answer cluster" <- w7
  "i ref out" <- w3
  "error out" <- w2
